vi "FRCts20_EspEngine_SetClosedEventRequestVariables.vi"(8 "error in (no error)":errorcluster, 10 "ClosedRequests":T1(array[cluster]), 11 "httpRequestID in":u32) -> (0 "error out":errorcluster, 3 "httpRequestID out":u32)   [LabVIEW 2014, in "FRCts20_EspEngine.lvlib"]
uses:
  FRCts20_EspEngine.lvlib
  <vilib>/wsapi/subVIs/Set Integer ESP Variable.vi
  FRCts20_EspEngine_FormatArrayOfKeysInts.vi
  FRCts20_EspEngine_FormatArrayOfKeysStrings.vi
  <vilib>/wsapi/NI_WebServices.lvlib
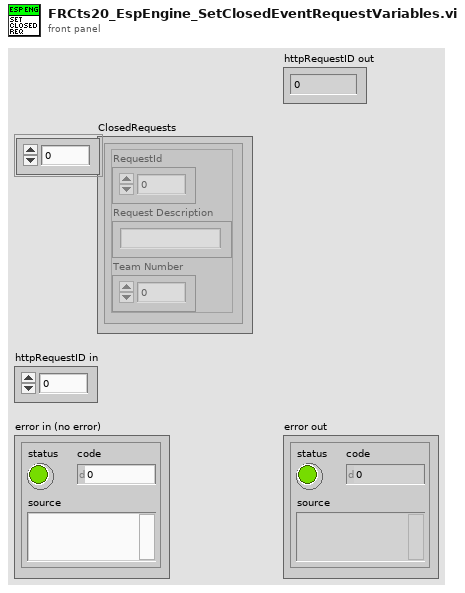
[diagram p1: front panel]
types:
  T1 = cluster{"RequestId":i32, "Request Description":string, "Team Number":i32}[]
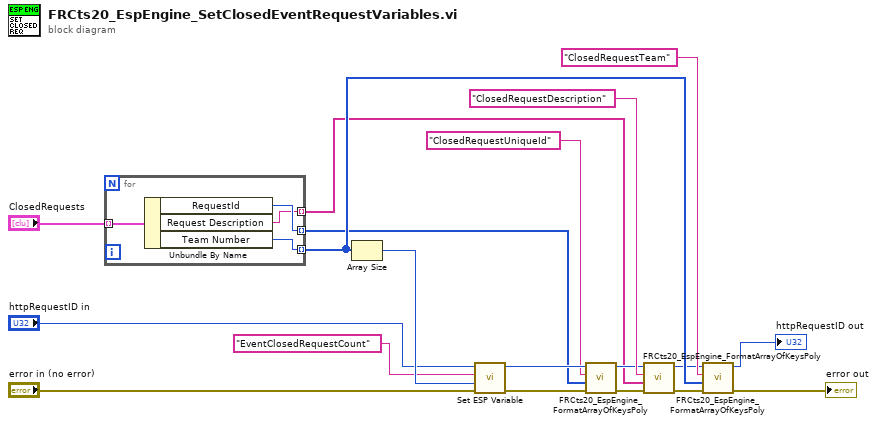
[diagram p0: block diagram]
diagram:
  n1 = for {
    tunnel: "ClosedRequests" -> [w23] mode=indexing
    tunnel: [w22] -> w7 mode=indexing
    tunnel: [w21] -> w4 mode=indexing
    tunnel: [w20] -> w14 mode=indexing
    n2 = Unbundle By Name(w23) -> ("RequestId"=w22:i32, "Request Description"=w21:string, "Team Number"=w20:i32)
  }
  n3 = Array Size(array=w14) -> (size(s)=w15:i32)
  n4 = call-poly <vilib>:"Set ESP Variable.vi"("error in (no error)"="error in (no error)", "value"=w15, "key"="EventClosedRequestCount", "httpRequestID"="httpRequestID in") -> ("error out"=w16:errorcluster, "httpRequestID out"=w17:u32)  [unwired: 6 in]
  n5 = call-poly "FRCts20_EspEngine_FormatArrayOfKeysPoly.vi"("error IO"=w16, "Values"=w7, "KeyBaseName"="ClosedRequestUniqueId", "httpRequestID"=w17) -> ("error IO"=w5:errorcluster, "httpRequestID out"=w8:u32)  [unwired: 6 in]
  n6 = call-poly "FRCts20_EspEngine_FormatArrayOfKeysPoly.vi"("error IO"=w5, "Values"=w4, "KeyBaseName"="ClosedRequestDescription", "httpRequestID"=w8) -> ("error IO"=w6:errorcluster, "httpRequestID out"=w9:u32)  [unwired: 6 in]
  n7 = call-poly "FRCts20_EspEngine_FormatArrayOfKeysPoly.vi"("error IO"=w6, "Values"=w14, "KeyBaseName"="ClosedRequestTeam", "httpRequestID"=w9) -> ("error IO"=→"error out":errorcluster, "httpRequestID out"=→"httpRequestID out":u32)  [unwired: 6 in]
